vi "BuildSequenceFile - XML.vi"(10 "Sequence File Data":T1, 11 "Sequence Context In":refnum<k7>) -> (0 "error out":errorcluster, 3 "NewSequenceFile":refnum<k7>)   [LabVIEW 2011]
doc: "This VI demonstrates how to cast a SequenceFile object in order access properties of the PropertyObjectFile and PropertyObject parent classes"
uses:
  HelperVIs.llb/SequenceFileData.ctl
  HelperVIs.llb/SequenceData.ctl
  HelperVIs.llb/StepGroup.ctl
  HelperVIs.llb/StepData.ctl
  HelperVIs.llb/StepProperties.ctl
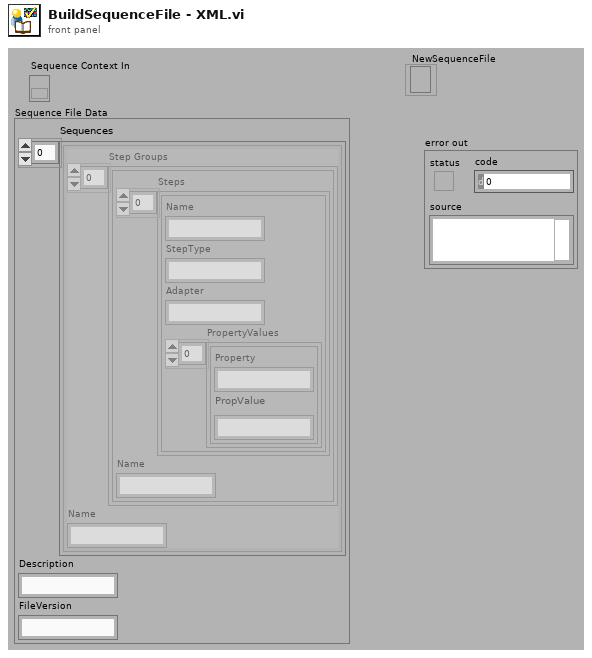
[diagram p1: front panel]
types:
  T1 = typedef "SequenceFileData.ctl" = cluster{"Sequences":T2[], "Description":string, "FileVersion":string}
  T2 = typedef "SequenceData.ctl" = cluster{"Step Groups":T3[], "Name":string}
  T3 = typedef "StepGroup.ctl" = cluster{"Steps":T4[], "Name":string}
  T4 = typedef "StepData.ctl" = cluster{"Name":string, "StepType":string, "Adapter":string, "PropertyValues":T5[]}
  T5 = typedef "StepProperties.ctl" = cluster{"Property":string, "PropValue":string}
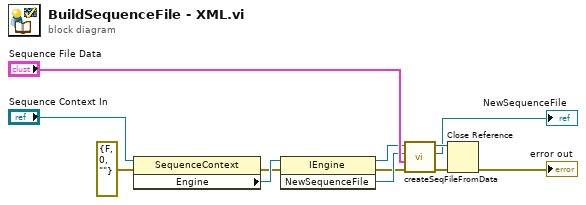
[diagram p0: block diagram]
diagram:
  n1 = property class="SequenceContext"(reference="Sequence Context In", error in=errorcluster {"status"=FALSE, "code"=0, "source"=""} ("error in (no error)")) -> (error out=w9:errorcluster, "Engine"=w12:refnum<k7>)  [unwired: 1 out]
  n2 = invoke class="IEngine" method="NewSequenceFile"(reference=w12, error in=w9) -> (reference out=w4:refnum<k7>, error out=w5:errorcluster, "NewSequenceFile"=w6:refnum<k7>)  [unwired: 1 in]
  n3 = call "createSeqFileFromData.vi"("error In"=w5, "Sequence File Data"="Sequence File Data", "NewSequenceFile"=w6, "Engine"=w4) -> ("error out"=w3:errorcluster, "NewSequenceFile"=→"NewSequenceFile":refnum<k7>, "Engine out"=w2:refnum<k7>)  [unwired: 5 in]
  n4 = Close Reference(reference=w2, error in (no error)=w3) -> (error out=→"error out":errorcluster)
